vi "lvEtherbone.handler_detach.vi"(0 "eb_socketID":i32, 1 "eb_handlerID":i32, 5 "error in (no error)":errorcluster) -> (13 "eb_status":T1, 14 "eb_socketID out":i32, 19 "error out":errorcluster)   [LabVIEW 2009, in "lvEtherbone.lvlib"]
doc: "//-----------------------------------------------------------------------------------\n// author : Dietrich Beck, GSI-Darmstadt\n// purpose : Detach the device from the virtual bus.\n// returns : lveb_status_t\n//-----------------------------------------------------------------------------------\nETHERBONE_API int lveb_handler_detach(int eb_handlerID //ID of handler\n );"
uses:
  lvEtherbone.lvlib
  lvEtherbone.lveb_status_t.ctl
  bin/lvEtherbone.dll
panel:
  in  "myeb_status_t":T1
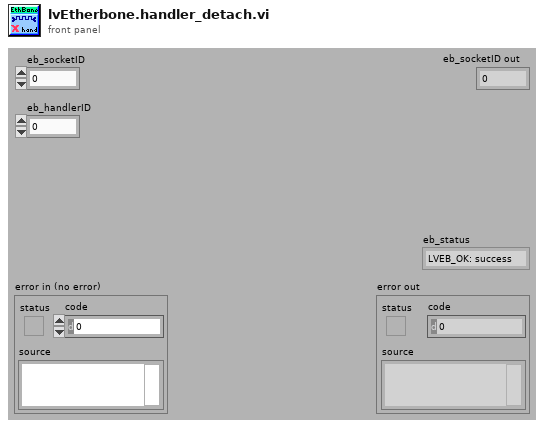
[diagram p1: front panel]
types:
  T1 = typedef "lvEtherbone.lvlib/lvEtherbone.lveb_status_t.ctl" = enum32{"LVEB_OK: success", "LVEB_UNKNOWN: unknown error", "LVEB_OS: operating system forbids access", "LVEB_PORT: port in use or unavailable", "LVEB_ID: ID invalid or out of resources", "LVEB_SOCKET: socket invalid or unavailable", "LVEB_EB: remote address is not Etherbone conformant", "LVEB_IP: bad format or network address", "LVEB_PORTWIDTH: port width error", "LVEB_DEVICEBUSY: Etherbone device still busy", "LVEB_DEVICEFAIL: operation on Wishbone device failed", "LVEB_DEVICEEXIST: Etherbone device already exists, overlaps, or does not exist", "LVEB_TIMEDOUT: a timeout occurred", "LVEB_OVERFLOW: payload of Etherbone exceeded", "LVEB_ADDRESS: bad address", "LVEB_ADDRESSWIDTH: address width error"}
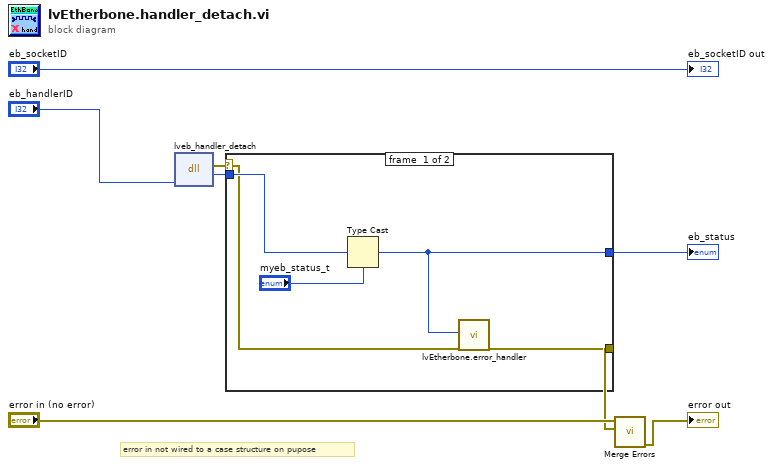
[diagram p0: block diagram]
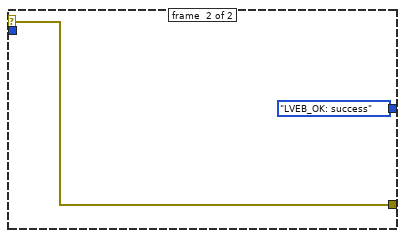
[diagram p2: hidden frame]
diagram:
  # "error in not wired to a case structure on pupose"
  n1 = dll-call lib="F:/beck/Project/BEL/SCC/etherbone-core/api/lvEtherbone/bin/lvEtherbone.*" fn="lveb_handler_detach"("eb_handlerID"="eb_handlerID") -> (error out=w5:errorcluster, "myeb_status"=w4:i32)  [unwired: 4 in, 1 out]
  n2 = case shown="No Error" w5 {
    selector: w5 -> [w9 w15]
    tunnel: w4 -> [w13 _]
    tunnel: [w11 lvEtherbone.lveb_status_t."LVEB_OK: success" ("eb_status_t")] -> w3
    tunnel: [w10 w15] -> w2
    frame #0 {
      n3 = Type Cast(type="myeb_status_t", x=w13) -> (*(type *) &x=w11:T1)
      n4 = call "lvEtherbone.error_handler.vi"("eb_status"=w11, "error in"=w9) -> ("error out"=w10:errorcluster)  [unwired: 17 in]
    }
    frame #1 {
    }
  }
  "eb_status" <- w3
  n5 = call <vilib>:"Merge Errors.vi"("error in 2 (no error)"=w2, "error in 1 (no error)"="error in (no error)") -> ("error out"=→"error out":errorcluster)  [unwired: 5 in]
  "eb_socketID out" <- "eb_socketID"
